vi "Seq Dialog Motion.vi"(6 "Segment Data":T4) -> (0 "Step Hisitory":string[](array[string]), 2 "Segment Data 2":T4)   [LabVIEW 2018]
uses:
  type defs/17x AP Data Type.ctl
  type defs/Sequence Info.ctl
  type defs/17x Audit Motion Data Seq Control.ctl
panel:
  in  "SW Mode":enum16{"Hard Switch", "Uncond Frame"}(ring)
  in  "LIN Msg":T1={"ID"=0, "Msg"=[], "LDF"="EX1H"} {"Msg" format="%02x"; "ID" format="%02x"}
  in  "Max Sound (dB)":dbl
  in  "Min Sound (dB)":dbl
  in  "Check Sound":bool
  in  "Check max Current":bool
  in  "Max max Current (amps)":dbl=10.0
  in  "Min max Current (amps)":dbl=10.0
  out "value":T2={"Power Supply Voltage"=0.0, "Min Avg Current"=0.0, "Max Avg Current"=0.0, "Min Run Time"=0.0, "Max Run Time"=0.0, "Min Speed"=0.0, "Max Speed"=0.0, "AP Data % of Threshold"=10.0, "Travel Distance"=0.0, "AP Data Type"=enum."91/61", "Check Current"=FALSE, "Check Run Time"=FALSE, "Check Speed"=FALSE, "Express Motion?"=FALSE, "Check Sound Test"=FALSE, "Check Position?"=FALSE, "Collect AP Data"=FALSE, "Inital Position"=0, "End Position"=0, "Goto Posiition"=0, "Max max Current"=0.0, "Min max Current"=0.0, "Check max Current"=FALSE, "Check Sound"=FALSE, "Min Sound (dB)"=0.0, "Max Sound (dB)"=0.0, "SW Mode"=enum."Hard Switch", "LIN Msg"={"ID"=0, "Msg"=[], "LDF"="EX1H"}} {"LIN Msg"."Msg" format="%02x"; "LIN Msg"."ID" format="%02x"}
  in  "Goto Position":u16=133
  in  "End Position":u16=133 format="%02x"
  in  "Initial Position":u16=133 format="%02x"
  in  "Max Speed (mm/sec)":dbl=10.0
  in  "Min Speed (mm/sec)":dbl=10.0
  in  "AP Data Type":T3
  in  "Check Position":bool
  in  "Express Motion":bool
  in  "Check Speed":bool
  in  "Travel Distance (mm)":dbl=133.0
  in  "Check Current":bool
  in  "Check Run Time":bool
  out "error out":errorcluster
  in  "Max Run Time (secs)":dbl=10.0
  in  "Min Run Time (secs)":dbl=10.0
  in  "Max Avg Current (amps)":dbl=10.0
  in  "Min Avg Current (amps)":dbl=10.0
  in  "Collect AP Data":bool
  in  "AP Data % of Threshold":dbl=80.0
  in  "Check Noise":bool
  in  "Description":string
  in  "Cancel":bool
  in  "Save":bool
  in  "PS Voltage (V)":dbl=13.0
  out "String":string="Pre Run Station - Glass - Vent Open"
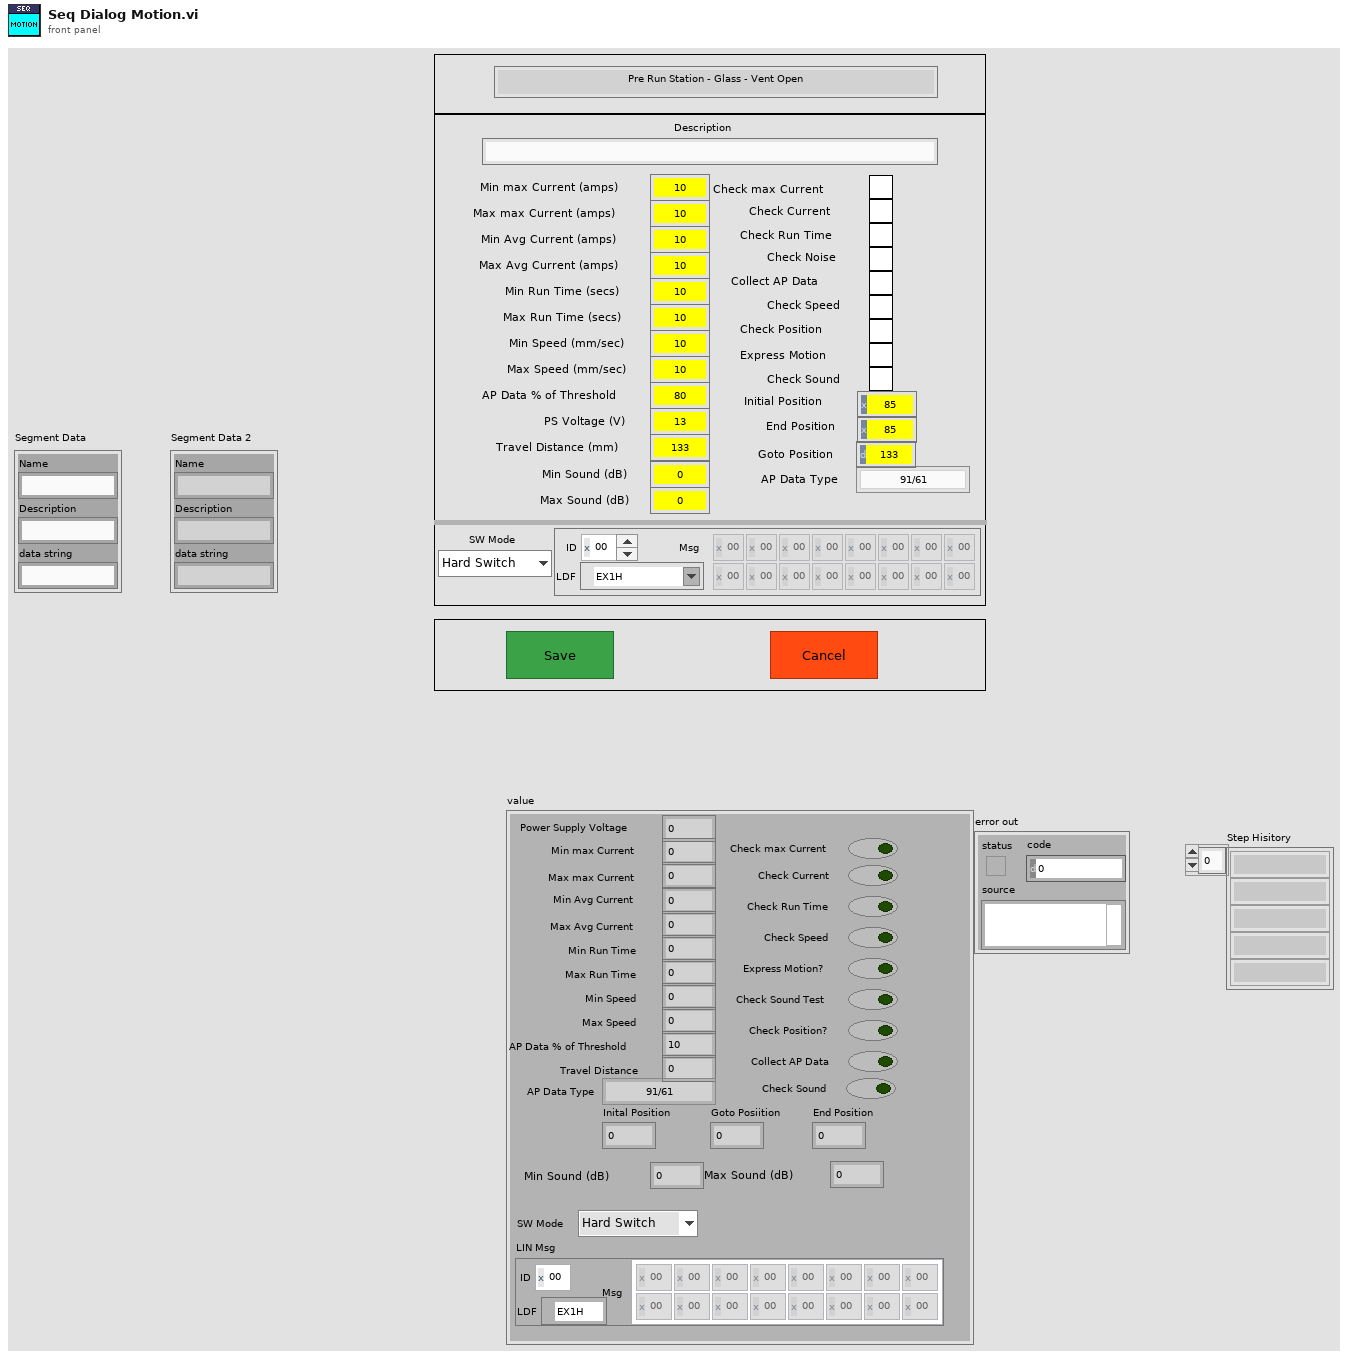
[diagram p1: front panel]
types:
  T1 = cluster{"ID":u8, "Msg":u8[][], "LDF":refnum<k21>}
  T2 = typedef "17x Audit Motion Data Seq Control.ctl" = cluster{"Power Supply Voltage":dbl, "Min Avg Current":dbl, "Max Avg Current":dbl, "Min Run Time":dbl, "Max Run Time":dbl, "Min Speed":dbl, "Max Speed":dbl, "AP Data % of Threshold":dbl, "Travel Distance":dbl, "AP Data Type":T3, "Check Current":bool, "Check Run Time":bool, "Check Speed":bool, "Express Motion?":bool, "Check Sound Test":bool, "Check Position?":bool, "Collect AP Data":bool, "Inital Position":u16, "End Position":u16, "Goto Posiition":u16, "Max max Current":dbl, "Min max Current":dbl, "Check max Current":bool, "Check Sound":bool, "Min Sound (dB)":dbl, "Max Sound (dB)":dbl, "SW Mode":enum16{"Hard Switch", "Uncond Frame"}, "LIN Msg":cluster{"ID":u8, "Msg":u8[][], "LDF":refnum<k21>}}
  T3 = typedef "17x AP Data Type.ctl" = enum16{"91/61", "92/62", "93/63", "67", "68", "6F", "71", "91 Msg", "92 Msg", "93 Msg", "94 Msg", "HiRain 91", "HiRain 92 Speed", "HiRain 92 HS", "HiRain 92", "HiRain 93", "SnT"}
  T4 = typedef "Sequence Info.ctl" = cluster{"Name":string, "Description":string, "data string":string}
  T5 = cluster{"Motion Data Cluster":T2, "Segment Data":T4, "Old Data":string, "New Data":string}
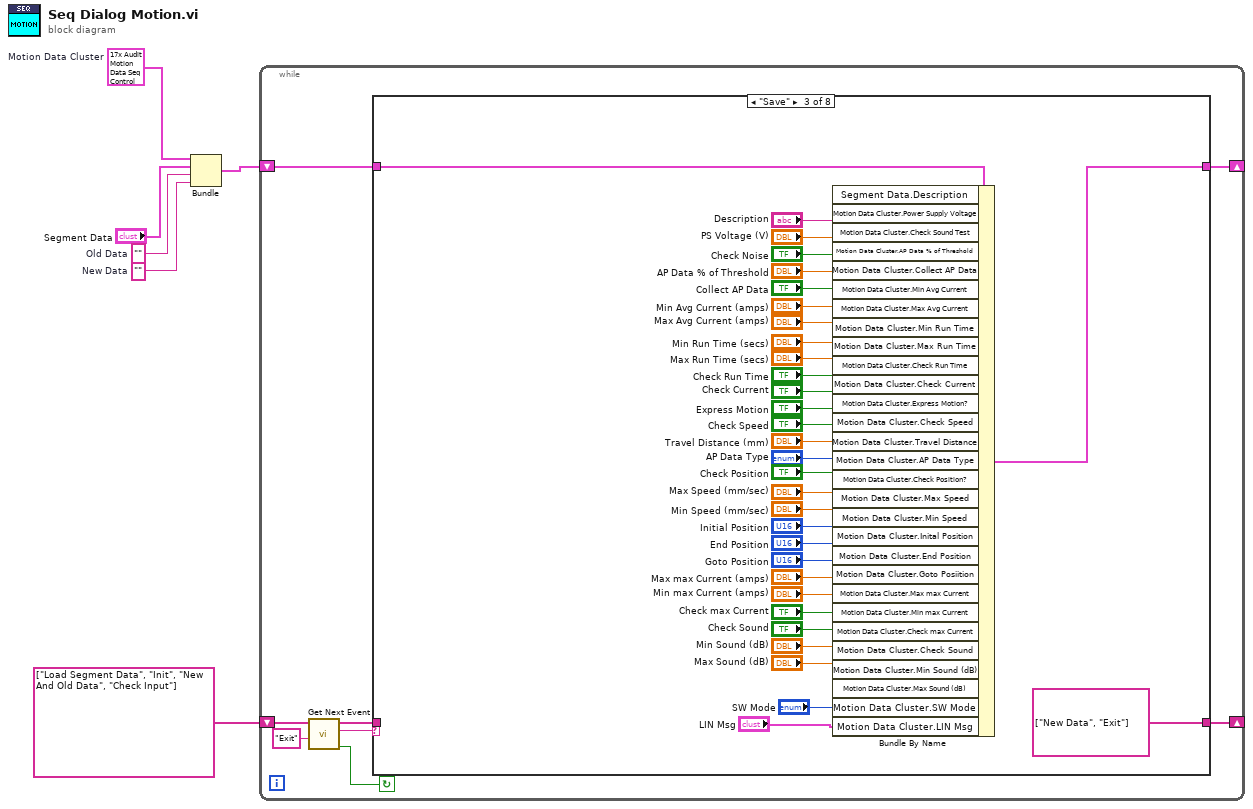
[diagram p0: block diagram]
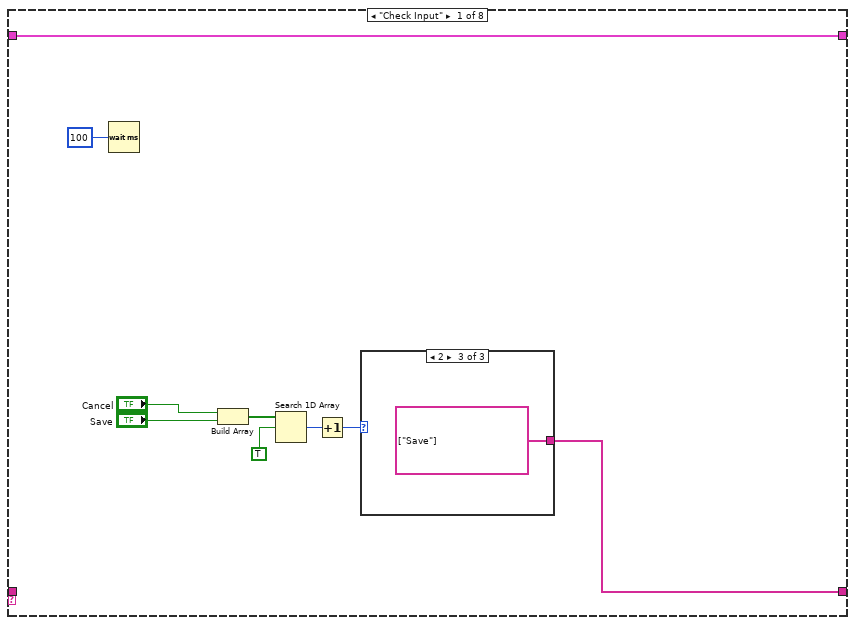
[diagram p2: hidden frame]
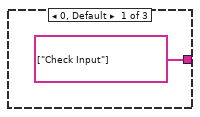
[diagram p3: hidden frame]
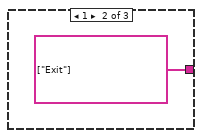
[diagram p4: hidden frame]
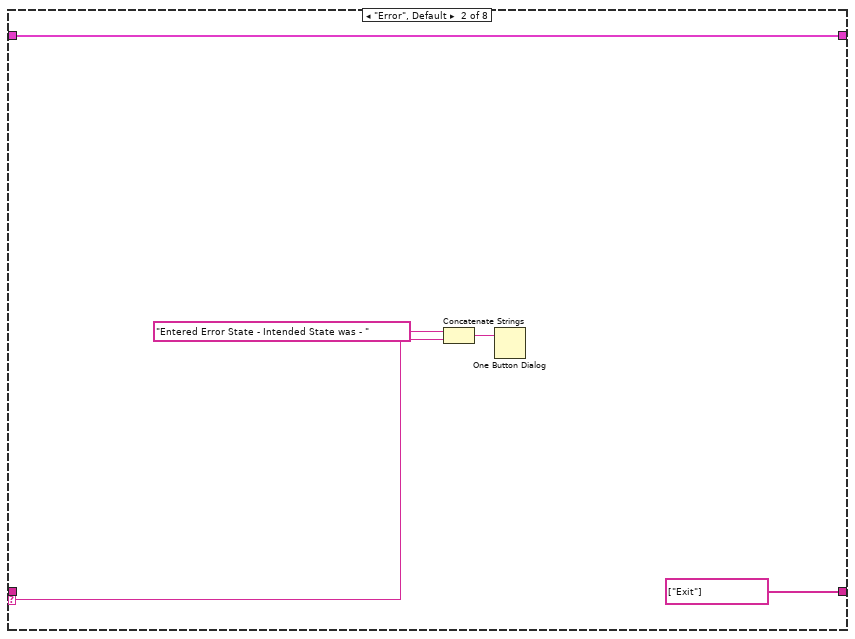
[diagram p5: hidden frame]
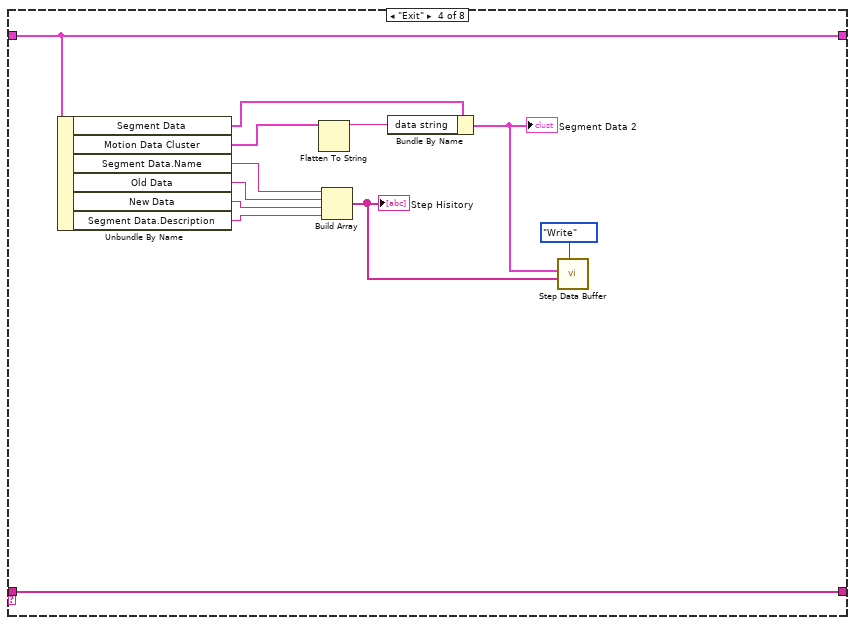
[diagram p6: hidden frame]
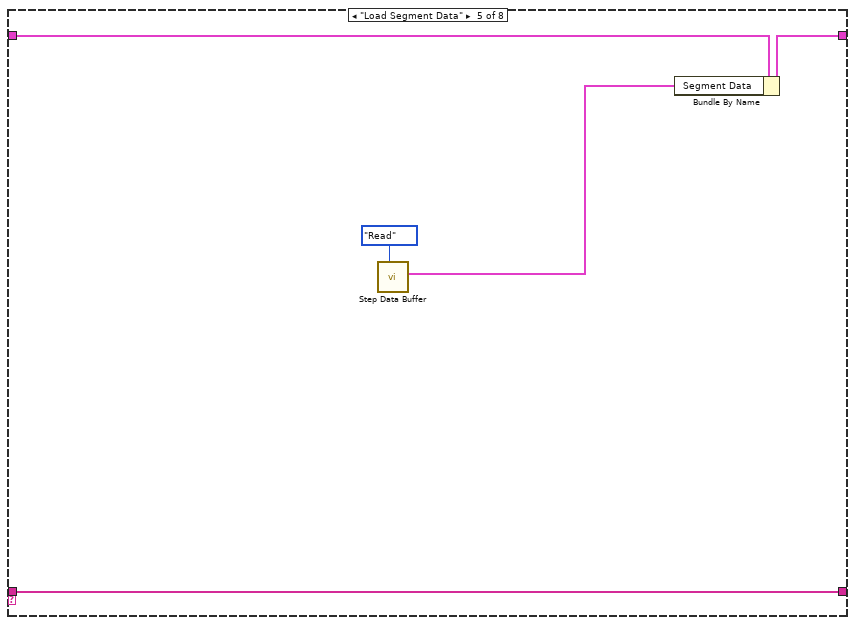
[diagram p7: hidden frame]
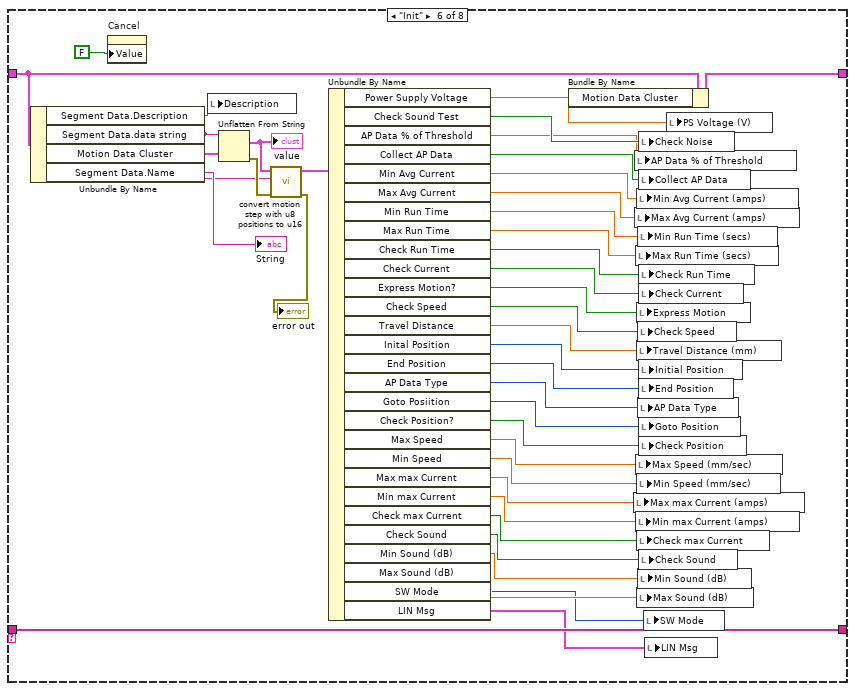
[diagram p8: hidden frame]
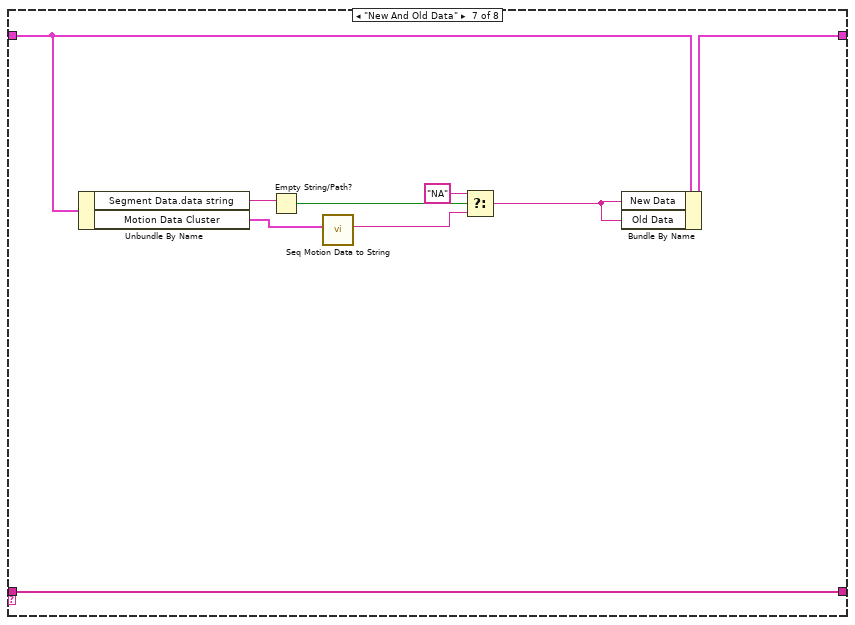
[diagram p9: hidden frame]
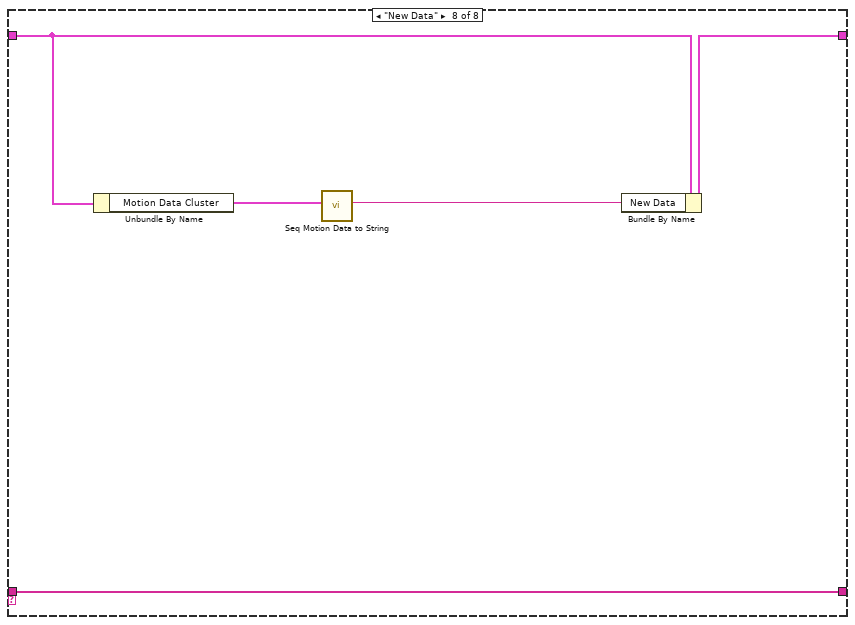
[diagram p10: hidden frame]
diagram:
  w2 = ""  # New Data
  w3 = ""  # Old Data
  w5 = T2 {"Power Supply Voltage"=0.0, "Min Avg Current"=0.0, "Max Avg Current"=0.0, "Min Run Time"=0.0, "Max Run Time"=0.0, "Min Speed"=0.0, "Max Speed"=0.0, "AP Data % of Threshold"=0.0, "Travel Distance"=0.0, "AP Data Type"=enum."91/61", "Check Current"=FALSE, "Check Run Time"=FALSE, "Check Speed"=FALSE, "Express Motion?"=FALSE, "Check Sound Test"=FALSE, "Check Position?"=FALSE, "Collect AP Data"=FALSE, "Inital Position"=0, "End Position"=0, "Goto Posiition"=0, "Max max Current"=0.0, "Min max Current"=0.0, "Check max Current"=FALSE, "Check Sound"=FALSE, "Min Sound (dB)"=0.0, "Max Sound (dB)"=0.0, "SW Mode"=enum."Hard Switch", "LIN Msg"={"ID"=0, "Msg"=[], "LDF"="EX1H"}}  # Motion Data Cluster
  n1 = Bundle("Motion Data Cluster"=w5, "Segment Data"="Segment Data", "Old Data"=w3, "New Data"=w2) -> (w6:T5)  [unwired: 1 in]
  n2 = while {
    shift-right: [w12] -> _
    shift-left: string[] ["Load Segment Data", "Init", "New And Old Data", "Check Input"] ("Event queue out") -> [w11]
    shift-right: [w7] -> _
    shift-left: w6 -> [w8]
    stop <- w10 continue-if-true
    n3 = call "Get Next Event.vi"("Exit Event"="Exit", "event queue in"=w11) -> ("Condition (Exit:F)"=w10:bool, "next event"=w14:string, "event queue out"=w13:string[])  [unwired: 3 in]
    n4 = case shown="\"Save\"" w14 {
      selector: w14 -> [_ w28 _ _ _ _ _ _]
      tunnel: w13 -> [_ _ _ w75 w79 w119 w129 w134]
      tunnel: [w17 string[] ["Exit"] ("event queue out") string[] ["New Data", "Exit"] ("Event queue out") w75 w79 w119 w129 w134] -> w12
      tunnel: w8 -> [w23 w27 w63 w71 w78 w117 w124 w133]
      tunnel: [w23 w27 w62 w71 w77 w116 w123 w132] -> w7
      frame "Check Input" {
        n5 = Wait (ms)(milliseconds to wait=u32 100) -> ()  [unwired: 1 out]
        n6 = Build Array("Cancel", "Save") -> (w19:bool[])
        n7 = Search 1D Array(1D array=w19, element=TRUE) -> (index of element=w20:i32)  [unwired: 1 in]
        n8 = Increment(x=w20) -> (x+1=w21:i32)
        n9 = case shown="2" w21 {
          tunnel: [string[] ["Check Input"] ("Events to Insert") string[] ["Exit"] ("Events to Insert") string[] ["Save"] ("Events to Insert")] -> w17
          frame 0, Default {
          }
          frame 1 {
          }
          frame 2 {
          }
        }
      }
      frame "Error", Default {
        n10 = Concatenate Strings("Entered Error State - Intended State was - " ("string"), w28) -> (w30:string)
        n11 = One Button Dialog(message=w30) -> ()  [unwired: 1 in, 1 out]
      }
      frame "Save" {
        n12 = Bundle By Name(cluster=w63, "Segment Data.Description"="Description", "Motion Data Cluster.Power Supply Voltage"="PS Voltage (V)", "Motion Data Cluster.Check Sound Test"="Check Noise", "Motion Data Cluster.AP Data % of Threshold"="AP Data % of Threshold", "Motion Data Cluster.Collect AP Data"="Collect AP Data", "Motion Data Cluster.Min Avg Current"="Min Avg Current (amps)", "Motion Data Cluster.Max Avg Current"="Max Avg Current (amps)", "Motion Data Cluster.Min Run Time"="Min Run Time (secs)", "Motion Data Cluster.Max Run Time"="Max Run Time (secs)", "Motion Data Cluster.Check Run Time"="Check Run Time", "Motion Data Cluster.Check Current"="Check Current", "Motion Data Cluster.Express Motion?"="Express Motion", "Motion Data Cluster.Check Speed"="Check Speed", "Motion Data Cluster.Travel Distance"="Travel Distance (mm)", "Motion Data Cluster.AP Data Type"="AP Data Type", "Motion Data Cluster.Check Position?"="Check Position", "Motion Data Cluster.Max Speed"="Max Speed (mm/sec)", "Motion Data Cluster.Min Speed"="Min Speed (mm/sec)", "Motion Data Cluster.Inital Position"="Initial Position", "Motion Data Cluster.End Position"="End Position", "Motion Data Cluster.Goto Posiition"="Goto Position", "Motion Data Cluster.Max max Current"="Max max Current (amps)", "Motion Data Cluster.Min max Current"="Min max Current (amps)", "Motion Data Cluster.Check max Current"="Check max Current", "Motion Data Cluster.Check Sound"="Check Sound", "Motion Data Cluster.Min Sound (dB)"="Min Sound (dB)", "Motion Data Cluster.Max Sound (dB)"="Max Sound (dB)", "Motion Data Cluster.SW Mode"="SW Mode", "Motion Data Cluster.LIN Msg"="LIN Msg") -> (w62:T5)
      }
      frame "Exit" {
        n13 = Unbundle By Name(w71) -> ("Segment Data"=w69:T4, "Motion Data Cluster"=w70:T2, "Segment Data.Name"=w73:string, "Old Data"=w72:string, "New Data"=w74:string, "Segment Data.Description"=w64:string)
        n14 = Flatten To String(anything=w70) -> (data string=w68:string)  [unwired: 3 in, 2 out]
        n15 = Build Array(w73, w72, w74, w64) -> (w65:string[])
        "Step Hisitory" <- w65
        n16 = Bundle By Name(cluster=w69, "data string"=w68) -> (w66:T4)
        "Segment Data 2" <- w66
        n17 = call "Step Data Buffer.vi"("Mode"=enum16{"Init", "Read", "Write"}."Write", "Step Hisitory In"=w65, "Segment Data In"=w66) -> ()  [unwired: 4 in, 5 out]
      }
      frame "Load Segment Data" {
        n18 = call "Step Data Buffer.vi"("Mode"=enum16{"Init", "Read", "Write"}."Read") -> ("Segment Data Out"=w76:T4)  [unwired: 6 in, 4 out]
        n19 = Bundle By Name(cluster=w78, "Segment Data"=w76) -> (w77:T5)
      }
      frame "Init" {
        n20 = Unbundle By Name(w117) -> ("Segment Data.Description"=w118:string, "Segment Data.data string"=w91:string, "Motion Data Cluster"=w120:T2, "Segment Data.Name"=→"String":string)
        n21 = property on="Cancel" class="Bool (严格)"("Value"=FALSE ("Cancel")) -> ()  [unwired: 2 in, 2 out]
        n22 = local write "Description"(w118) -> ()
        n23 = Unflatten From String(type=w120, binary string=w91) -> (value=w90:T2, error out=w93:errorcluster)  [unwired: 3 in, 1 out]
        "value" <- w90
        n24 = call "convert motion step with u8 positions to u16.vi"("error in"=w93, "data string"=w91, "Motion Data Cluster in"=w90) -> ("error out"=→"error out":errorcluster, "Motion Data Cluster out"=w89:T2)  [unwired: 7 in]
        n25 = Unbundle By Name(w89) -> ("Power Supply Voltage"=w115:dbl, "Check Sound Test"=w114:bool, "AP Data % of Threshold"=w113:dbl, "Collect AP Data"=w112:bool, "Min Avg Current"=w111:dbl, "Max Avg Current"=w110:dbl, "Min Run Time"=w109:dbl, "Max Run Time"=w108:dbl, "Check Run Time"=w107:bool, "Check Current"=w106:bool, "Express Motion?"=w105:bool, "Check Speed"=w104:bool, "Travel Distance"=w103:dbl, "Inital Position"=w101:u16, "End Position"=w100:u16, "AP Data Type"=w99:T3, "Goto Posiition"=w98:u16, "Check Position?"=w97:bool, "Max Speed"=w96:dbl, "Min Speed"=w95:dbl, "Max max Current"=w88:dbl, "Min max Current"=w87:dbl, "Check max Current"=w86:bool, "Check Sound"=w85:bool, "Min Sound (dB)"=w84:dbl, "Max Sound (dB)"=w83:dbl, "SW Mode"=w82:enum16{"Hard Switch", "Uncond Frame"}, "LIN Msg"=w81:T1)
        n26 = Bundle By Name(cluster=w117, "Motion Data Cluster"=w89) -> (w116:T5)
        n27 = local write "Max max Current (amps)"(w88) -> ()
        n28 = local write "AP Data % of Threshold"(w113) -> ()
        n29 = local write "Max Avg Current (amps)"(w110) -> ()
        n30 = local write "Max Run Time (secs)"(w108) -> ()
        n31 = local write "Max Speed (mm/sec)"(w96) -> ()
        n32 = local write "Min max Current (amps)"(w87) -> ()
        n33 = local write "Min Avg Current (amps)"(w111) -> ()
        n34 = local write "Express Motion"(w105) -> ()
        n35 = local write "Travel Distance (mm)"(w103) -> ()
        n36 = local write "Min Speed (mm/sec)"(w95) -> ()
        n37 = local write "Check max Current"(w86) -> ()
        n38 = local write "Max Sound (dB)"(w83) -> ()
        n39 = local write "Min Run Time (secs)"(w109) -> ()
        n40 = local write "Check Speed"(w104) -> ()
        n41 = local write "AP Data Type"(w99) -> ()
        n42 = local write "Min Sound (dB)"(w84) -> ()
        n43 = local write "Check Noise"(w114) -> ()
        n44 = local write "Collect AP Data"(w112) -> ()
        n45 = local write "Check Run Time"(w107) -> ()
        n46 = local write "Check Current"(w106) -> ()
        n47 = local write "Initial Position"(w101) -> ()
        n48 = local write "End Position"(w100) -> ()
        n49 = local write "Goto Position"(w98) -> ()
        n50 = local write "Check Position"(w97) -> ()
        n51 = local write "Check Sound"(w85) -> ()
        n52 = local write "SW Mode"(w82) -> ()
        n53 = local write "LIN Msg"(w81) -> ()
        n54 = local write "PS Voltage (V)"(w115) -> ()
      }
      frame "New And Old Data" {
        n55 = Unbundle By Name(w124) -> ("Segment Data.data string"=w128:string, "Motion Data Cluster"=w122:T2)
        n56 = Empty String/Path?(string/path=w128) -> (empty?=w127:bool)
        n57 = call "Seq Motion Data to String.vi"("Motion Data Cluster"=w122) -> ("Data String"=w121:string)  [unwired: 10 in]
        n58 = Select(t="NA", s=w127, f=w121) -> (s? t:f=w125:string)
        n59 = Bundle By Name(cluster=w124, "New Data"=w125, "Old Data"=w125) -> (w123:T5)
      }
      frame "New Data" {
        n60 = Unbundle By Name(w133) -> ("Motion Data Cluster"=w131:T2)
        n61 = call "Seq Motion Data to String.vi"("Motion Data Cluster"=w131) -> ("Data String"=w130:string)  [unwired: 10 in]
        n62 = Bundle By Name(cluster=w133, "New Data"=w130) -> (w132:T5)
      }
    }
  }
